vi "ccd_triggeredacquire_bkup.vi"() -> ()   [LabVIEW 2016]
panel:
  out "output path":path
  out "Y 3":dbl
  out "X 3":dbl
  out "Y 2":dbl
  out "X 2":dbl
  out "Image 2":T1(plugin-control)
  out "Image":T1(plugin-control)
  out "cameraName":dbl
  out "imageType":dbl
  out "trigger_number":dbl
  out "framenumber":dbl
  out "Y":dbl
  out "X":dbl
  in  "Trigger action":u32(ring)=1 items=["Disabled", "Trigger start of acquisition", "Trigger start of each buffer list", "Trigger each buffer", "Trigger each line (linescan)", "Trigger end of acquisition"]
  in  "Trigger Type":u32(ring) items=["External", "RTSI", "ISO In"]
  in  "Data frames / trigger":dbl=10.0
  in  "Video Frames / Data frame":dbl=15.0
  in  "GO":bool
  in  "stop":bool
  in  "Manual (up) or automatic (down)":bool
  in  "Or, read path automatically from:":path=path "\\\\Foghorn.bio.brandeis.edu\\remote"
  in  "Manual save directory":string
  in  "Manual save path":path
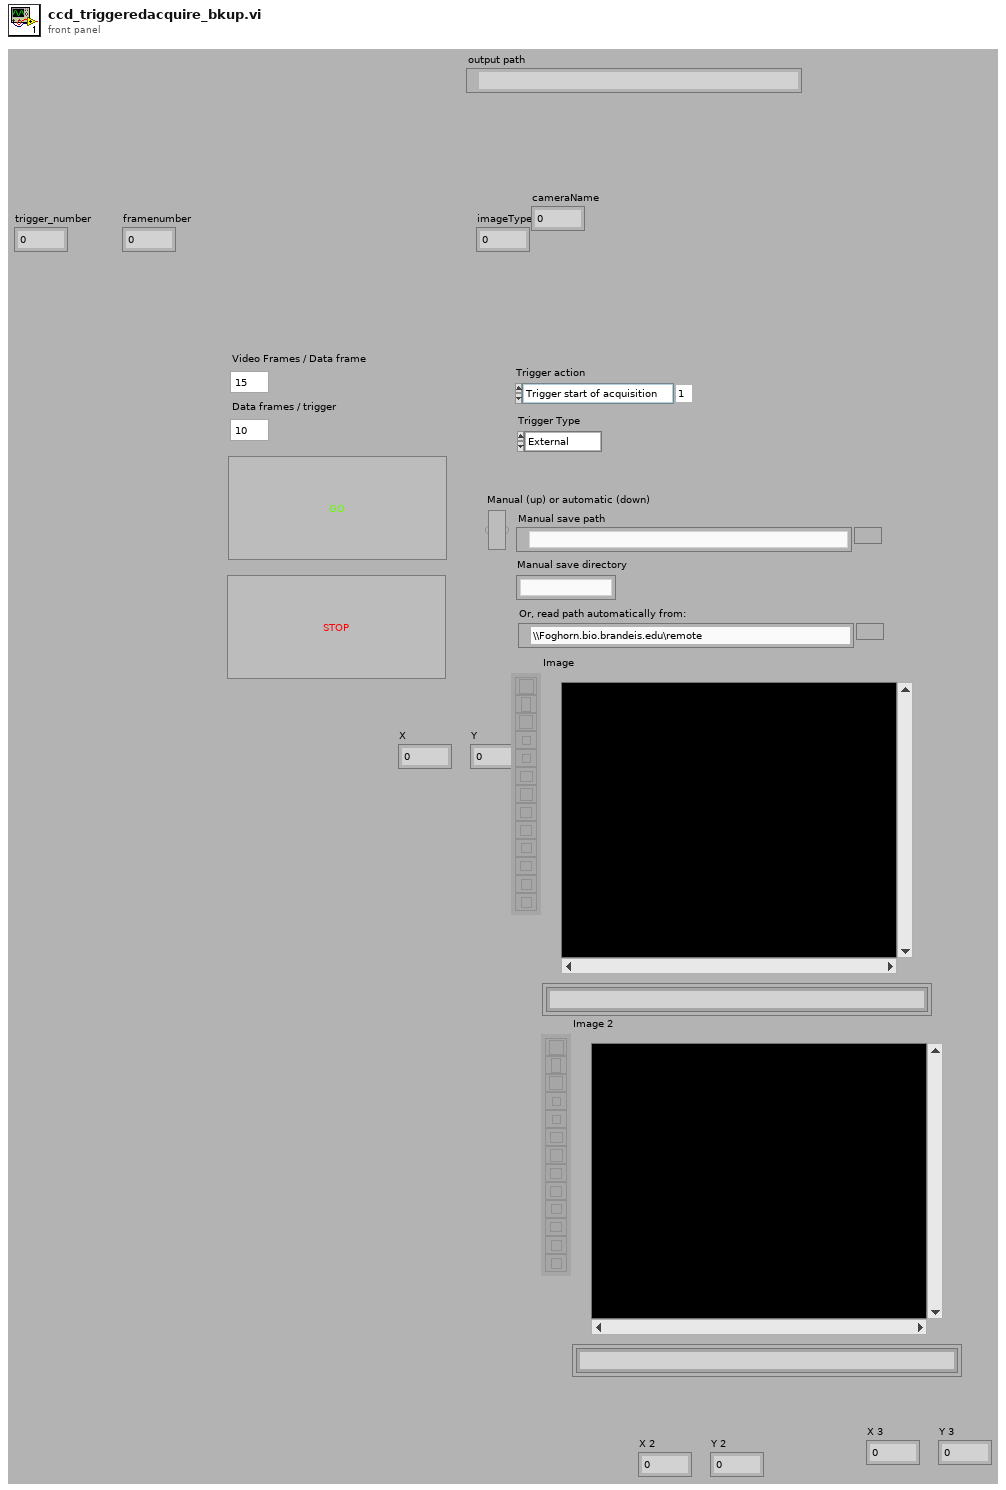
[diagram p1: front panel]
types:
  T1 = typedef "IMAQ Image.ctl" = refnum<image>
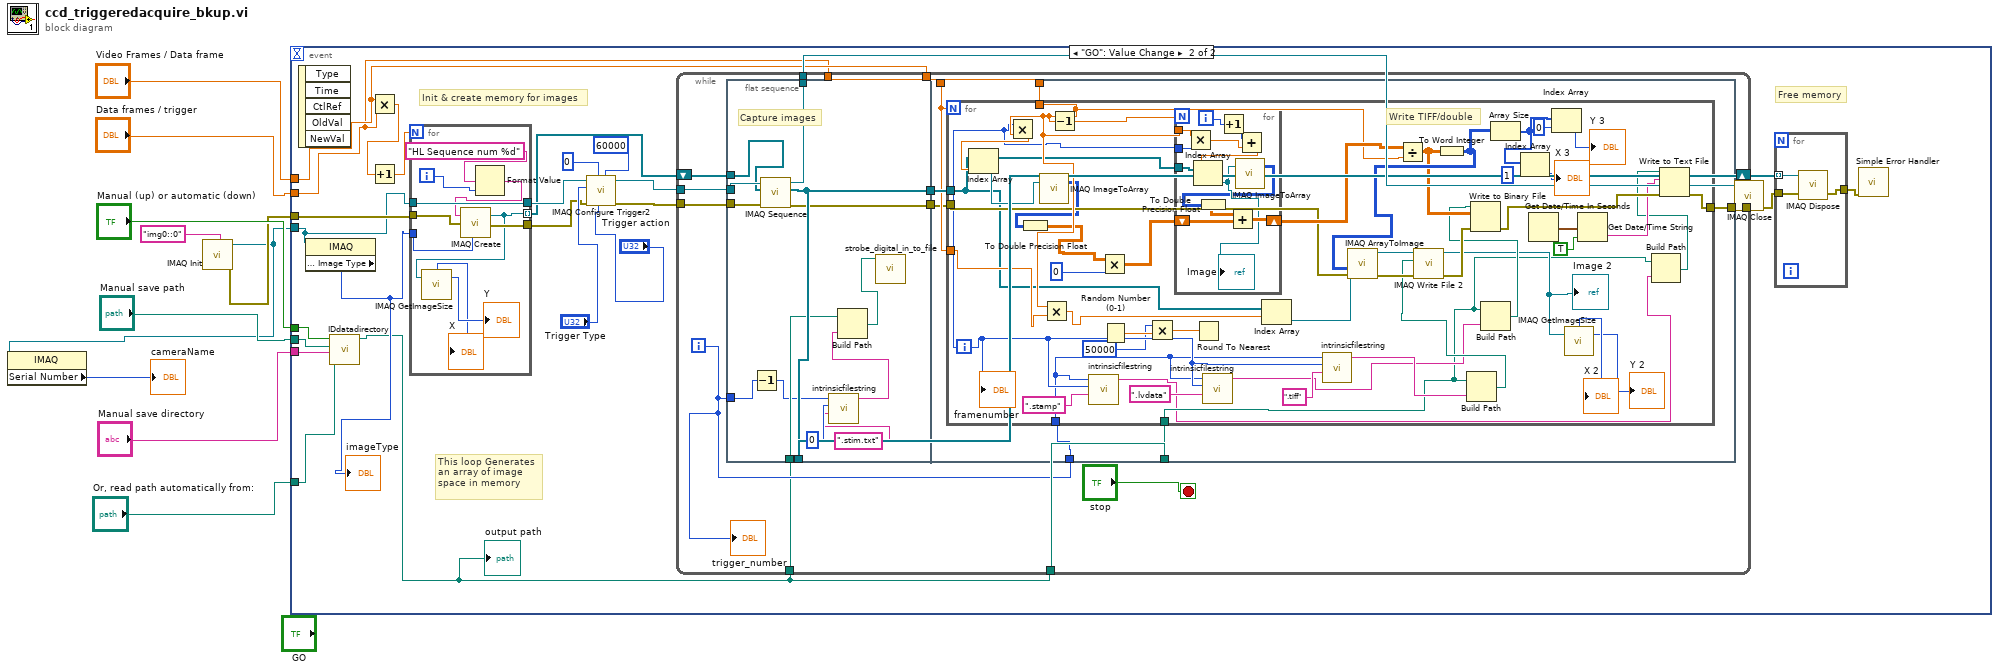
[diagram p0: block diagram]
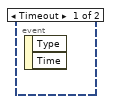
[diagram p2: hidden frame]
diagram:
  n1 = call <vilib>:"IMAQ Init.vi"("Interface Name"="img0::0") -> ("error out"=w4:errorcluster, "IMAQ Session Out"=w2:refnum<k11>)  [unwired: 9 in]
  n2 = property class="IMAQ"(reference=w2) -> ("Serial Number"=→"cameraName":u32)  [unwired: 1 in, 2 out]
  n3 = event shown="[1] \"GO\": Value Change" {
    selector: _ -> [_ _]
    dyn-events: _ -> [_ _]
    timeout: _ -> [_ _]
    tunnel: "Video Frames / Data frame" -> [_ w23]
    tunnel: "Data frames / trigger" -> [_ w22]
    tunnel: "Or, read path automatically from:" -> [_ w27]
    tunnel: "Manual save directory" -> [_ w26]
    tunnel: "Manual save path" -> [_ w25]
    tunnel: "Manual (up) or automatic (down)" -> [_ w24]
    tunnel: w4 -> [_ w15]
    tunnel: w2 -> [_ w14]
    event Timeout {
      n4 = event-data() -> ()  [unwired: 1 in, 2 out]
    }
    event "GO": Value Change {
      # "Free memory"
      # "This loop Generates an array of image space in memory"
      # "Init & create memory for images"
      n5 = event-data() -> ()  [unwired: 1 in, 5 out]
      n6 = property class="IMAQ"(reference=w14) -> ("Image Parameters : Image Type"=w13:u32)  [unwired: 1 in, 2 out]
      "imageType" <- w13
      n7 = call "IDdatadirectory.vi"("Read path automatically from:"=w27, "Directory"=w26, "Save path"=w25, "Manual or automatic"=w24) -> ("Outputpath"=w11:path)  [unwired: 7 in]
      "output path" <- w11
      n8 = Multiply(x=w23, y=w22) -> (x*y=w21:dbl)
      n9 = Increment(x=w21) -> (x+1=w20:dbl)
      n10 = for {
        N: w20 -> [_]
        tunnel: [w142] -> w32
        tunnel: [w138] -> w19 mode=indexing
        tunnel: w15 -> [w141]
        tunnel: w14 -> [w140]
        tunnel: [w140] -> w33
        tunnel: w13 -> [w139]
        i -> [w134]
        n11 = Format Value(format string="HL Sequence num %d", value (0)=w134) -> (output string=w133:string)  [unwired: 1 in]
        n12 = call "IMAQ Create"("Image Name"=w133, "Image Type"=w139, "error in (no error)"=w141) -> ("New Image"=w138:T1, "error out"=w142:errorcluster)  [unwired: 2 in]
        n13 = call "IMAQ GetImageSize"("Image"=w138) -> ("Y Resolution"=→"Y":i32, "X Resolution"=→"X":i32)  [unwired: 3 in, 1 out]
      }
      n14 = call <vilib>:"IMAQ Configure Trigger2.vi"("Frame timeout (ms)"=u32 60000, "Trigger action"="Trigger action", "Trigger Polarity"=0, "error in (no error)"=w32, "Trigger Type"="Trigger Type", "IMAQ Session In"=w33) -> ("error out"=w30:errorcluster, "IMAQ Session Out"=w31:refnum<k11>)  [unwired: 4 in]
      n15 = while {
        tunnel: w31 -> [w53]
        tunnel: w30 -> [w52]
        shift-right: [w45] -> w18
        shift-left: w19 -> [w47]
        tunnel: [w50] -> w28
        tunnel: w11 -> [w42]
        tunnel: w23 -> [w49]
        tunnel: w22 -> [w48]
        tunnel: [w43] -> w17
        tunnel: w11 -> [w40]
        i -> [w41]
        stop <- "stop" stop-if-true
        n16 = flat-sequence {
          tunnel: w53 -> [w64]
          tunnel: w52 -> [w66]
          tunnel: [w62] -> w51
          tunnel: [w65] -> w50
          tunnel: w47 -> [w63]
          tunnel: [w62] -> w45
          tunnel: [w61] -> w44
          tunnel: w41 -> [w55]
          tunnel: w40 -> [w56]
          tunnel: w51 -> [w73]
          tunnel: w42 -> [w72]
          tunnel: w41 -> [w67]
          tunnel: w49 -> [w71]
          tunnel: w48 -> [w70]
          tunnel: w44 -> [w69]
          tunnel: [w68] -> w43
          frame #0 {
            # "Capture images"
            n17 = Decrement(x=w55) -> (x-1=w54:i32)
            n18 = call <vilib>:"IMAQ Sequence.vi"("error in (no error)"=w66, "Images In"=w63, "IMAQ Session In"=w64) -> ("error out"=w61:errorcluster, "Images Out"=w62:T1[], "IMAQ Session Out"=w65:refnum<k11>)  [unwired: 6 in]
            n19 = call "intrinsicfilestring.vi"("Postfix"=".stim.txt", "Frame number"=0, "Trigger number"=w54) -> ("Filestring"=w57:string)  [unwired: 8 in]
            n20 = Build Path(base path=w56, name or relative path=w57) -> (appended path=w60:path)
            n21 = call "strobe_digital_in_to_file.vi"("Path"=w60) -> ()  [unwired: 11 in]
          }
          frame #1 {
            n22 = for {
              N: w70 -> [_]
              tunnel: w73 -> [w79]
              tunnel: w72 -> [w89]
              tunnel: w67 -> [w75]
              tunnel: w71 -> [w115]
              tunnel: w70 -> [w117]
              tunnel: w69 -> [w113]
              tunnel: [w87] -> w68
              i -> [w90]
              # "Write TIFF/double"
              n23 = Multiply(x=w90, y=w115) -> (x*y=w119:dbl)
              n24 = Index Array(array=w79, index=w119) -> (element=w120:T1)
              n25 = call "IMAQ ImageToArray"("Image"=w120) -> ("Image Pixels (I16)"=w103:i16[][])  [unwired: 3 in, 4 out]
              n26 = To Double Precision Float(number=w103) -> (double precision float=w78:dbl[][])
              n27 = Multiply(x=w115, y=w117) -> (x*y=w114:dbl)
              n28 = Decrement(x=w115) -> (x-1=w118:dbl)
              n29 = call "intrinsicfilestring.vi"("Postfix"=".stamp", "Frame number"=w90, "Trigger number"=w75) -> ("Filestring"=w88:string)  [unwired: 8 in]
              n30 = Multiply(x=w78, y=0) -> (x*y=w77:dbl[][])
              n31 = Random Number (0-1)() -> (number: 0 to 1=w82:dbl)
              n32 = Multiply(x=50000, y=w82) -> (x*y=w80:dbl)
              n33 = for {
                N: w118 -> [_]
                tunnel: w79 -> [w132]
                shift-right: [w129] -> w116
                shift-left: w77 -> [w130]
                tunnel: w115 -> [w127]
                tunnel: w90 -> [w126]
                i -> [w128]
                n34 = Multiply(x=w127, y=w126) -> (x*y=w124:dbl)
                n35 = Increment(x=w128) -> (x+1=w125:i32)
                n36 = Add(x=w125, y=w124) -> (x+y=w123:dbl)
                n37 = Index Array(array=w132, index=w123) -> (element=w122:T1)
                "Image" <- w122
                n38 = call "IMAQ ImageToArray"("Image"=w122) -> ("Image Pixels (I16)"=w121:i16[][])  [unwired: 3 in, 4 out]
                n39 = To Double Precision Float(number=w121) -> (double precision float=w131:dbl[][])
                n40 = Add(x=w131, y=w130) -> (x+y=w129:dbl[][])
              }
              n41 = Round To Nearest(number=w80) -> ()  [unwired: 1 out]
              n42 = call "intrinsicfilestring.vi"("Postfix"=".lvdata", "Frame number"=w90, "Trigger number"=w75) -> ("Filestring"=w94:string)  [unwired: 8 in]
              n43 = Index Array(array=w79, index=w114) -> (element=w99:T1)
              n44 = call "intrinsicfilestring.vi"("Postfix"=".tiff", "Frame number"=w90, "Trigger number"=w75) -> ("Filestring"=w101:string)  [unwired: 8 in]
              n45 = Divide(x=w116, y=w115) -> (x/y=w95:dbl[][])
              n46 = To Word Integer(number=w95) -> (16bit integer=w102:i16[][])
              n47 = call "IMAQ ArrayToImage"("error in (no error)"=w113, "Image Pixels (I16)"=w102, "Image"=w99) -> ("error out"=w112:errorcluster, "Image Out"=w111:T1)  [unwired: 7 in]
              n48 = Build Path(base path=w89, name or relative path=w101) -> (appended path=w98:path)
              n49 = call-poly "IMAQ Write File 2"("error in (no error)"=w112, "File Path"=w98, "Image"=w111) -> ("error out"=w96:errorcluster, "Image Out (duplicate)"=w92:T1)  [unwired: 7 in]
              "Image 2" <- w92
              n50 = Build Path(base path=w89, name or relative path=w94) -> (appended path=w93:path)
              n51 = Write to Binary File(file (use dialog)=w93, data=w95, error in=w96) -> (error out=w86:errorcluster)  [unwired: 3 in, 2 out]
              n52 = Array Size(array=w102) -> (size(s)=w107:i32[])
              n53 = Index Array(array=w107, index=1) -> (element=→"X 3":i32)
              n54 = Get Date/Time In Seconds() -> (seconds since 1Jan1904=w83:timestamp)
              n55 = Index Array(array=w107, index=0) -> (element=→"Y 3":i32)
              n56 = call "IMAQ GetImageSize"("Image"=w92) -> ("Y Resolution"=→"Y 2":i32, "X Resolution"=→"X 2":i32)  [unwired: 3 in, 1 out]
              n57 = Get Date/Time String(seconds (now)=w83, want seconds? (F)=TRUE) -> (time string=w85:string)  [unwired: 1 in, 1 out]
              n58 = Build Path(base path=w89, name or relative path=w88) -> (appended path=w84:path)
              n59 = Write to Text File(file (use dialog)=w84, text=w85, error in=w86) -> (error out=w87:errorcluster)  [unwired: 1 in, 2 out]
              "framenumber" <- w90
            }
          }
        }
        "trigger_number" <- w41
      }
      n60 = call <vilib>:"IMAQ Close.vi"("error in (no error)"=w17, "IMAQ Session In"=w28) -> ("error out"=w16:errorcluster)  [unwired: 9 in]
      n61 = for {
        tunnel: w18 -> [w39] mode=indexing
        tunnel: w16 -> [w38]
        tunnel: [w37] -> w29
        n62 = call "IMAQ Dispose"("Image"=w39, "error in (no error)"=w38) -> ("error out"=w37:errorcluster)  [unwired: 4 in]
      }
      n63 = call <vilib>:"Simple Error Handler.vi"("error in (no error)"=w29) -> ()  [unwired: 4 in, 5 out]
    }
  }
